vi "popUpMain.vi"(8 "Error In":errorcluster, 10 "Message Description":string, 11 "Message Titlt":string) -> (0 "Error Out":errorcluster, 3 "Ok?":bool)   [LabVIEW 2018]
panel:
  in  "OK Button":bool
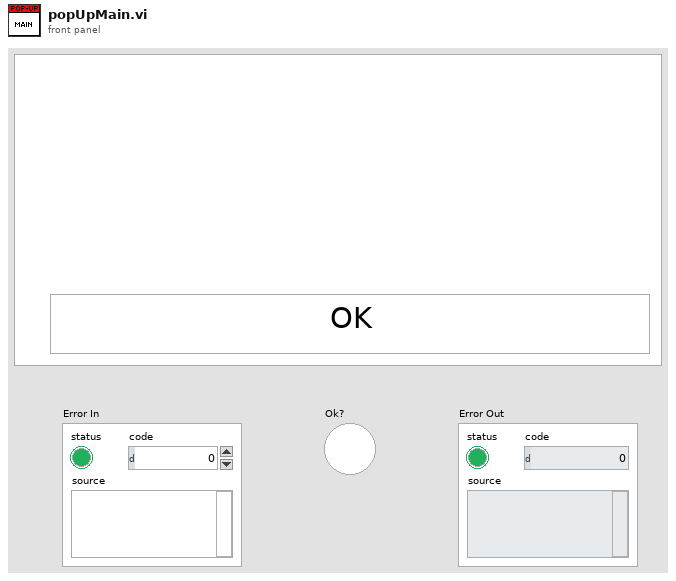
[diagram p1: front panel]
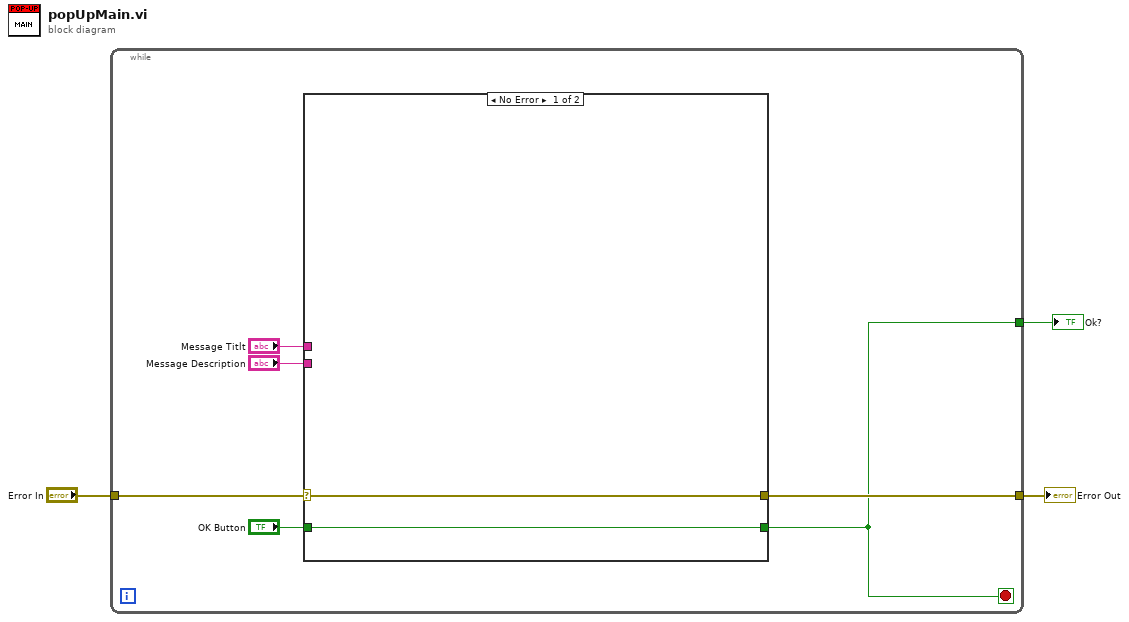
[diagram p0: block diagram]
diagram:
  n1 = while {
    tunnel: "Error In" -> [w9]
    tunnel: [w8] -> w2
    tunnel: [w4] -> w1
    stop <- w4 stop-if-true
    n2 = case shown="No Error" w9 {
      selector: w9 -> [w11 w13]
      tunnel: [w11 w13] -> w8
      tunnel: "Message Titlt" -> [_ _]
      tunnel: "Message Description" -> [_ _]
      tunnel: "OK Button" -> [w10 w12]
      tunnel: [w10 w12] -> w4
      frame No Error {
      }
      frame Error {
      }
    }
  }
  "Error Out" <- w2
  "Ok?" <- w1
